vi "HWhist-SingleCurve.vi"() -> ()   [LabVIEW 2023]
doc: "This example demonstrates how to use the Becker&Hickl LV wrappers to acquire single decay curves in a continuous loop.\nThe SPC parameters can be adjusted during the run. The rates and status flags are continuously updated.\nIt is also possible to save the acquired data to a SDT or CSV file.\nClick this window's red X to stop this VI.\n\ninfo@becker-hickl.com"
uses:
  SPC_Wrappers/SPC_Controls/ConfigMem.ctl
  Example_Controls/UserInput.ctl
  SPC_Wrappers/SPC_Controls/SPC_RatesCluster.ctl
  SPC_Wrappers/SPC_Controls/ADCResolution.ctl
  SPC_Wrappers/SPC_Controls/ModuleType.ctl
  SPC_Wrappers/SPC_Controls/SPCdata.ctl
  SPC_Wrappers/SPC_Controls/StateCluster.ctl
  SPC_Wrappers/SPC_Controls/dither_range.ctl
  SPC_Wrappers/SPC_Controls/macro_time_clk.ctl
  <vilib>/Utility/file.llb/Write Delimited Spreadsheet (I64).vi
panel:
  in  "Page":i16(ring) caption="Use Page No" items=["0", "1", "2", "3", "4", "5", "6", "7", "8", "9", "10", "11", "12", "13", "14", "15"]
  in  "Init":bool
  out "SPC_StateCluster":T1
  out "SPCdata":T2
  in  "TO":i32=-1
  in  "Module Type":T3=150 items=["SPC-600"=600, "SPC-630"=630, "SPC-700"=700, "SPC-730"=730, "SPC-130"=130, "SPC-830"=830, "SPC-140"=140, "SPC-930"=930, "DPC-230"=230, "SPC-150"=150, "SPC-150 N"=151, "SPC-150 NX"=152, "SPC-130 EM"=131, "SPC-130 EMN"=132, "SPC-130IN"=135, "SPC-130INX"=136, "SPC-130INXX"=137, "SPC-160"=160, "SPC-160 X"=161, "SPC-160 PCIE"=162, "SPC-180 N"=180, "SPC-180 NX"=181, "SPC-180 NXX"=182, "SPC-180 N-USB"=185, "SPC-180 NX-USB"=186, "SPC-180 NXX-USB"=187, "SPC-QC-104"=104, "SPC-QC-004"=4, "SPC-QC-106"=106, "DPC-330"=330, "PMS-800"=800, "SPC-590"=590, "Simulation"=-1]
  out "Serial Number":string="3F0668"
  in  "RepeatMeas":bool
  in  "SingleMeas":bool
  out "DLL Path":path=path "C:/Program Files (x86)/BH/SPCM/DLL/spcm32x64.dll"
  out "Data":u16[][](graph)
  in  "Save Data As":enum32{"SDT", "CSV"}(radio)
  in  "No of Routing Channels":i16(ring)=1 items=["1"=1, "2"=2, "3"=3, "4"=4, "5"=5, "6"=6, "7"=7, "8"=8, "9"=9, "10"=10, "11"=11, "12"=12, "13"=13, "14"=14, "15"=15, "16"=16]
  in  "ADC Resolution":T4=12 items=["1"=0, "4"=2, "16"=4, "64"=6, "256"=8, "1024"=10, "4096"=12]
  out "Mod No":i16
  out "Sync OK":bool=TRUE
  out "SPC_RatesCluster":T5={"Sync"=49999360.0, "CFD"=1709808.0, "TAC"=1444208.0, "ADC"=998080.0} {"Sync" scale=0.0..6000000.0; "ADC" scale=0.0..1000000.0; "TAC" scale=0.0..1000000.0; "CFD" scale=0.0..1000000.0}
  in  "User Input":T6={"tac_range"=50.0, "tac_gain"=3, "tac_offset"=12.0, "tac_limit_high"=96.0, "tac_limit_low"=3.0, "collect_time"=2.0, "sync_threshold"=-71.0, "sync_zc_level"=-5.0, "sync_freq_div"=1, "cfd_limit_low"=-50.0, "cfd_zc_level"=9.8} {"sync_freq_div" items=["1"=1, "2"=2, "4"=4]; "cfd_zc_level" min=-96 max=96 step=0.1 format="%#_3g"; "cfd_limit_low" min=-500 max=0 step=0.1 format="%#_3g"; "sync_zc_level" min=-96 max=96 step=0.1 format="%#_3g"; "sync_threshold" min=-500 max=-20 step=0.1 format="%#_3g"; "tac_limit_low" format="%.3g"; "tac_limit_high" min=0 max=100 step=0.1 format="%.3g"; "collect_time" min=1e-07 max=100000 step=0.001; "tac_offset" min=0 max=100 step=0.1 format="%.4g"; "tac_gain" min=1 max=15 step=1; "tac_range" format="%^#_6g"}
  in  "SaveData":bool
  in  "Name Of File":string="HW-SingleDecay"
  in  "SavingFolder":path=path "C:/temp"
  out "SPC memory config":T7={"Max Block No"=16384, "Blocks Per Frame"=1, "Frames Per Page"=1, "Maxpage"=16384, "Block Length"=256} {"Frames Per Page" min=1 step=1; "Maxpage" min=1; "Blocks Per Frame" min=1 step=1}
  in  "StopVi":bool=TRUE
  # "This example demonstrates how to use the Becker&Hickl LV wrappers to acquire single decay curves in a continuous loop.\nThe SPC parameters can be adjusted during the run. The rates and status flags are continuously updated.\nIt is also possible to save the acquired data to a SDT or CSV file.\nClick this window's red X to stop this VI."
  # "See Tip-Strip for details"
  # "(c) 2023 Becker & Hickl GmbH\n     ALL RIGHTS RESERVED."
  # "TAC / Time Range"
  # "CFD"
  # "(start)"
  # "SYNC"
  # "(stop)"
  # "range"
  # "gain"
  # "threshold(LL)"
  # "offset"
  # "limit high"
  # "limit low"
  # "zero cross(ZC)"
  # "Collection Time"
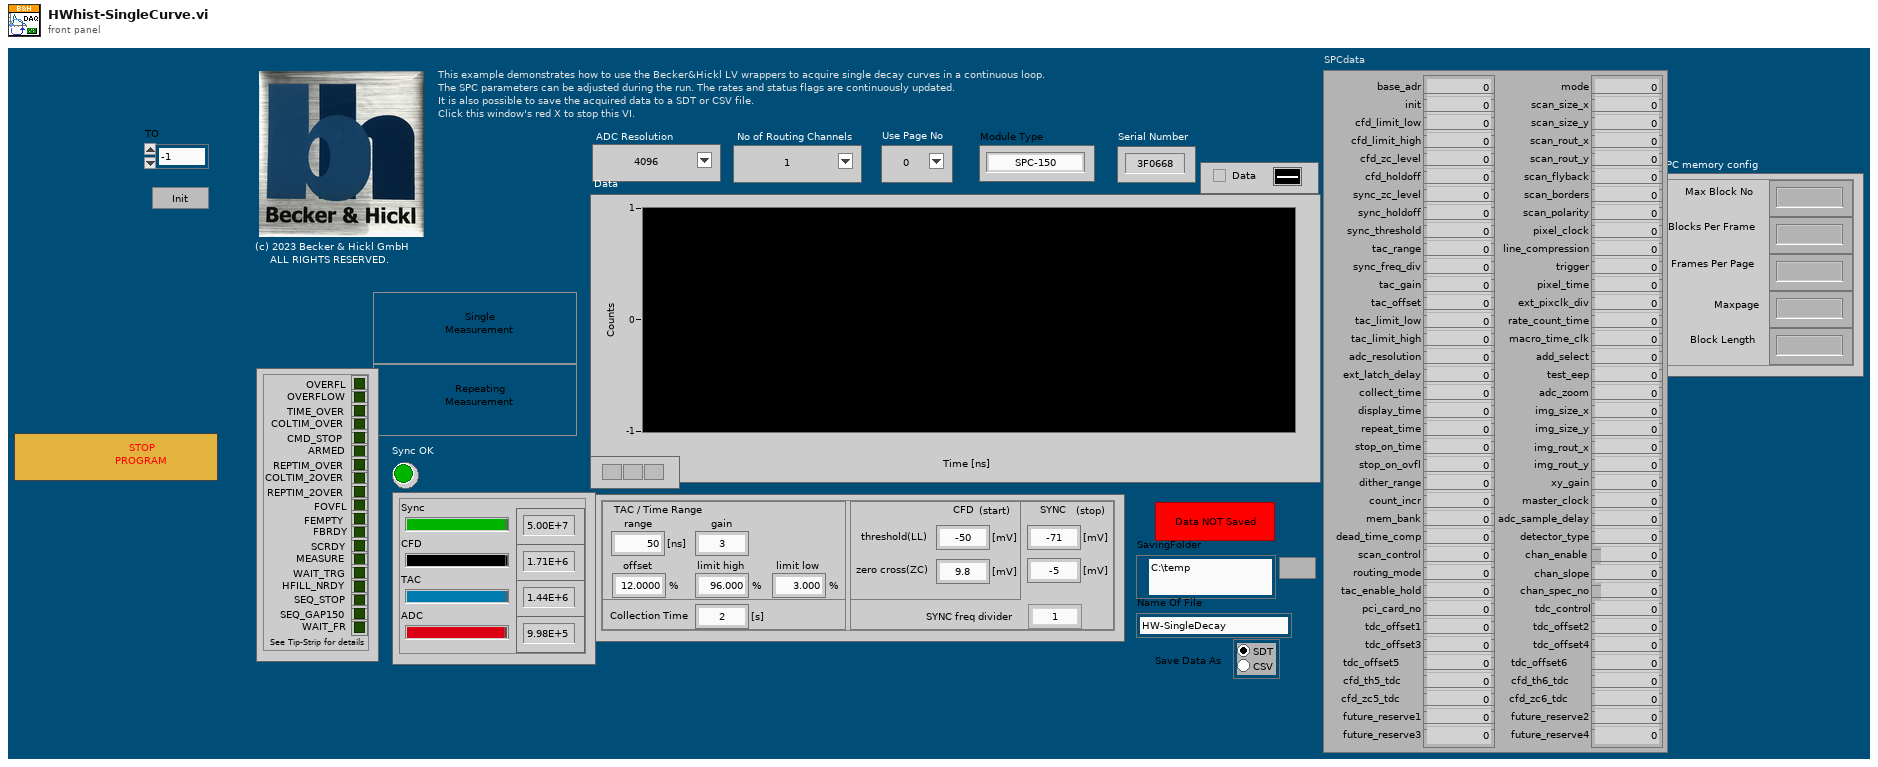
[diagram p1: front panel]
types:
  T1 = typedef "StateCluster.ctl" = cluster{"OVERFL":bool, "OVERFLOW":bool, "TIME_OVER":bool, "COLTIM_OVER":bool, "CMD_STOP":bool, "ARMED":bool, "REPTIM_OVER":bool, "COLTIM_2OVER":bool, "REPTIM_2OVER":bool, "FOVFL":bool, "FEMPTY":bool, "FBRDY":bool, "SCRDY":bool, "MEASURE":bool, "WAIT_TRG":bool, "HFILL_NRDY":bool, "SEQ_STOP":bool, "SEQ_GAP150":bool, "WAIT_FR":bool}
  T2 = typedef "SPCdata.ctl" = cluster{"base_adr":u16, "init":i16, "cfd_limit_low":sgl, "cfd_limit_high":sgl, "cfd_zc_level":sgl, "cfd_holdoff":sgl, "sync_zc_level":sgl, "sync_holdoff":sgl, "sync_threshold":sgl, "tac_range":sgl, "sync_freq_div":i16, "tac_gain":i16, "tac_offset":sgl, "tac_limit_low":sgl, "tac_limit_high":sgl, "adc_resolution":i16, "ext_latch_delay":i16, "collect_time":sgl, "display_time":sgl, "repeat_time":sgl, "stop_on_time":i16, "stop_on_ovfl":i16, "dither_range":i16, "count_incr":i16, "mem_bank":i16, "dead_time_comp":i16, "scan_control":u16, "routing_mode":u16, "tac_enable_hold":sgl, "pci_card_no":i16, "mode":u16, "scan_size_x":u32, "scan_size_y":u32, "scan_rout_x":u32, "scan_rout_y":u32, "scan_flyback":u32, "scan_borders":u32, "scan_polarity":u16, "pixel_clock":u16, "line_compression":u16, "trigger":u16, "pixel_time":sgl, "ext_pixclk_div":u32, "rate_count_time":sgl, "macro_time_clk":i16, "add_select":i16, "test_eep":i16, "adc_zoom":i16, "img_size_x":u32, "img_size_y":u32, "img_rout_x":u32, "img_rout_y":u32, "xy_gain":i16, "master_clock":i16, "adc_sample_delay":i16, "detector_type":i16, "chan_enable":u32, "chan_slope":u32, "chan_spec_no":u32, "tdc_control":u32, "tdc_offset1":sgl, "tdc_offset2":sgl, "tdc_offset3":sgl, "tdc_offset4":sgl, "tdc_offset5":sgl, "tdc_offset6":sgl, "cfd_th5_tdc":sgl, "cfd_th6_tdc":sgl, "cfd_zc5_tdc":sgl, "cfd_zc6_tdc":sgl, "future_reserve1":u64, "future_reserve2":u64, "future_reserve3":u64, "future_reserve4":u64}
  T3 = typedef "ModuleType.ctl" = i16
  T4 = typedef "ADCResolution.ctl" = i16
  T5 = typedef "SPC_RatesCluster.ctl" = cluster{"Sync":sgl, "CFD":sgl, "TAC":sgl, "ADC":sgl}
  T6 = typedef "UserInput.ctl" = cluster{"tac_range":sgl, "tac_gain":i16, "tac_offset":sgl, "tac_limit_high":sgl, "tac_limit_low":sgl, "collect_time":sgl, "sync_threshold":sgl, "sync_zc_level":sgl, "sync_freq_div":i16, "cfd_limit_low":sgl, "cfd_zc_level":sgl}
  T7 = typedef "ConfigMem.ctl" = cluster{"Max Block No":i32, "Blocks Per Frame":i32, "Frames Per Page":i32, "Maxpage":i32, "Block Length":i32}
  T8 = typedef "macro_time_clk.ctl" = enum16{"25ns", "Sync", "1/2 Sync", "1/4 Sync", "1/8 Sync"}
  T9 = typedef "dither_range.ctl" = i16
  T10 = enum8{"Enabled", "Disabled", "Disabled and Grayed Out"}
  T11 = typedef "SPCModInfo.ctl" = cluster{"Module Type":T3, "Bus Number":i16, "Slot Number":i16, "in Use":i16, "Init Status":i16, "Base I/O Addr":u16}
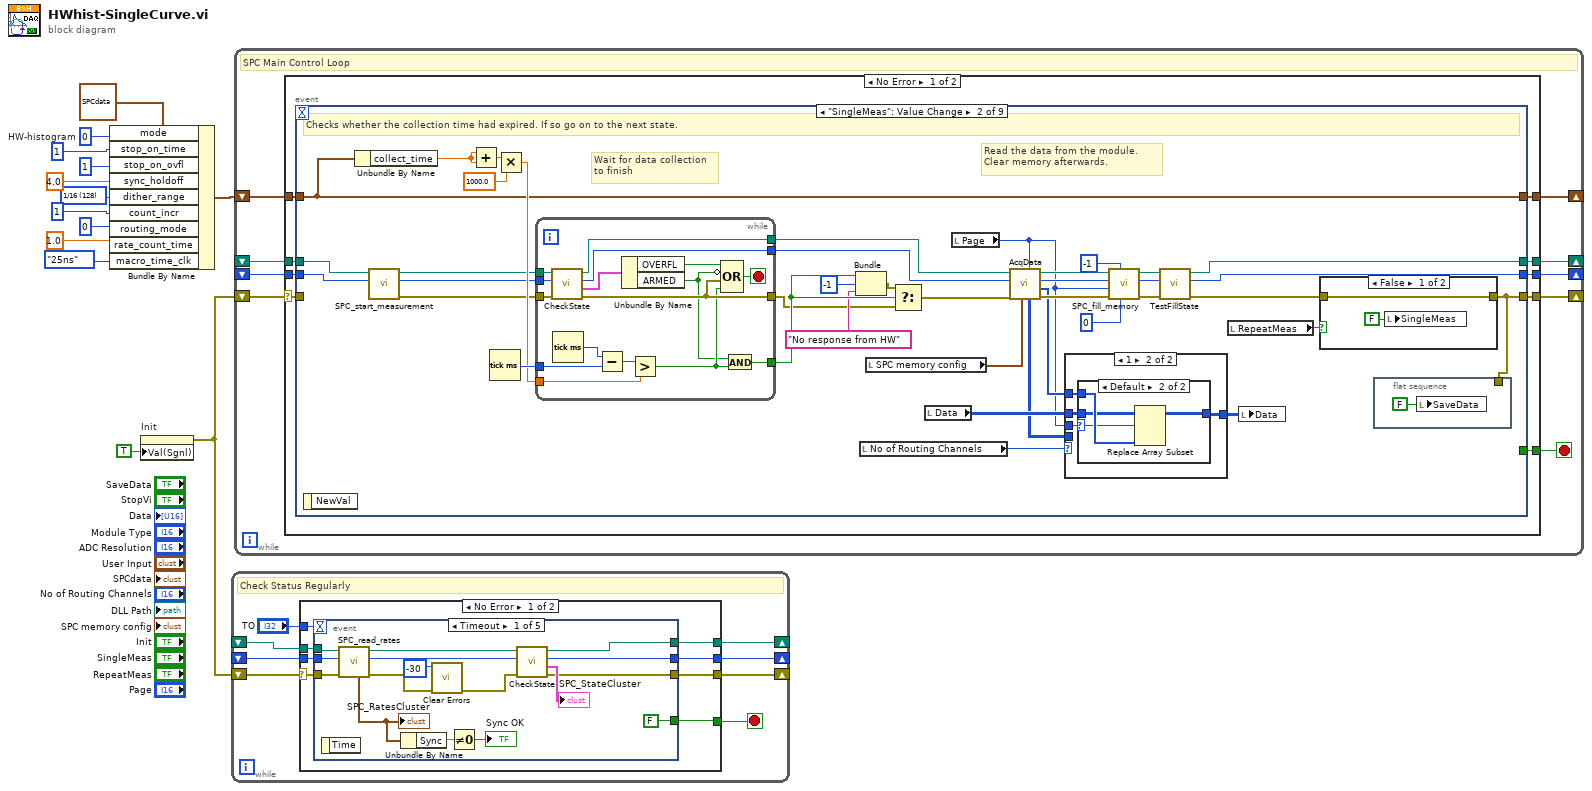
[diagram p0: block diagram]
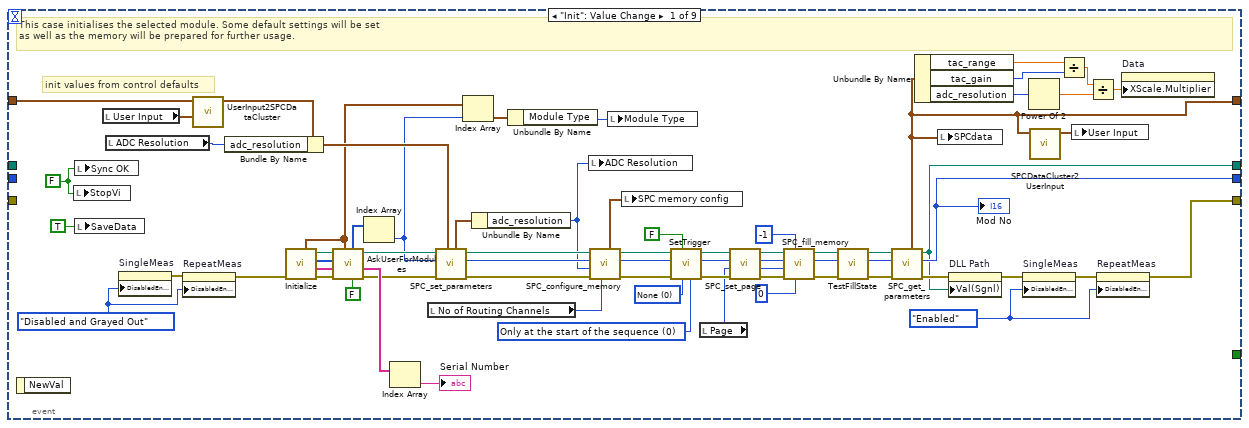
[diagram p2: hidden frame]
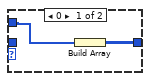
[diagram p4: hidden frame]
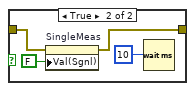
[diagram p5: hidden frame]
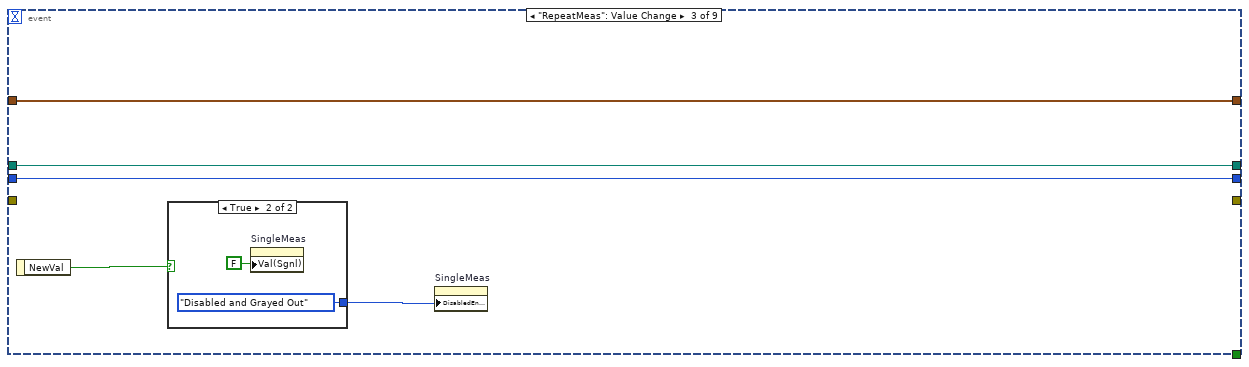
[diagram p6: hidden frame]
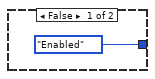
[diagram p7: hidden frame]
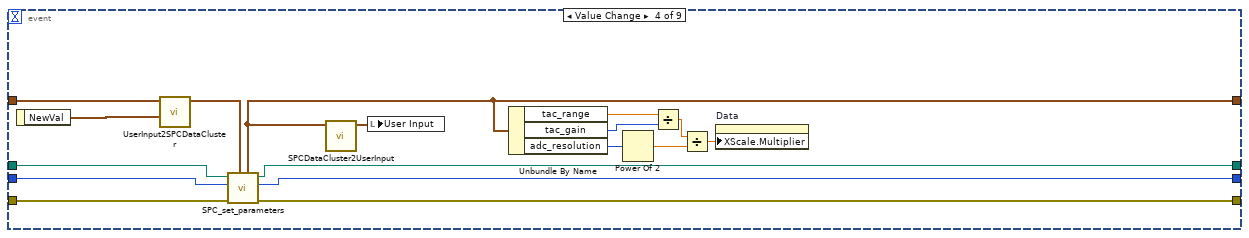
[diagram p8: hidden frame]
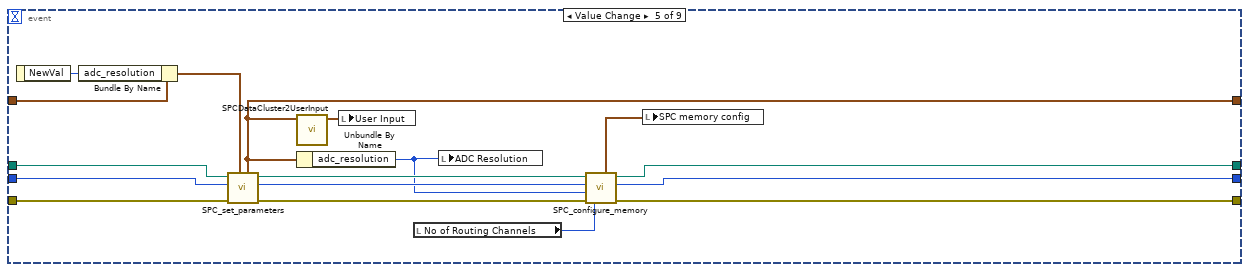
[diagram p9: hidden frame]
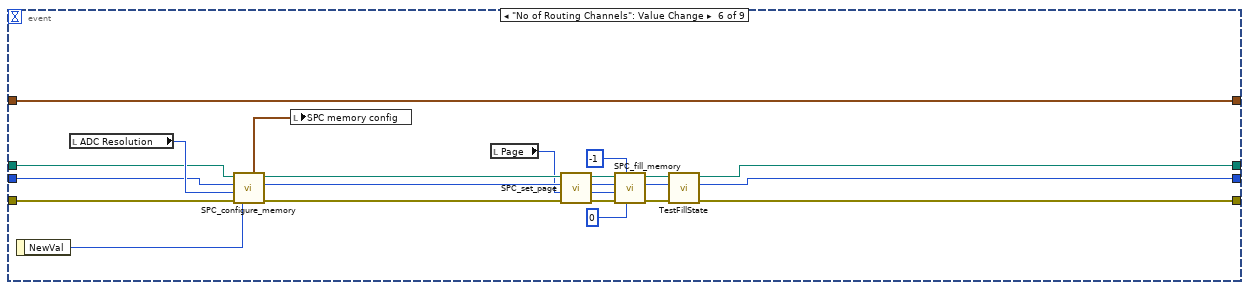
[diagram p10: hidden frame]
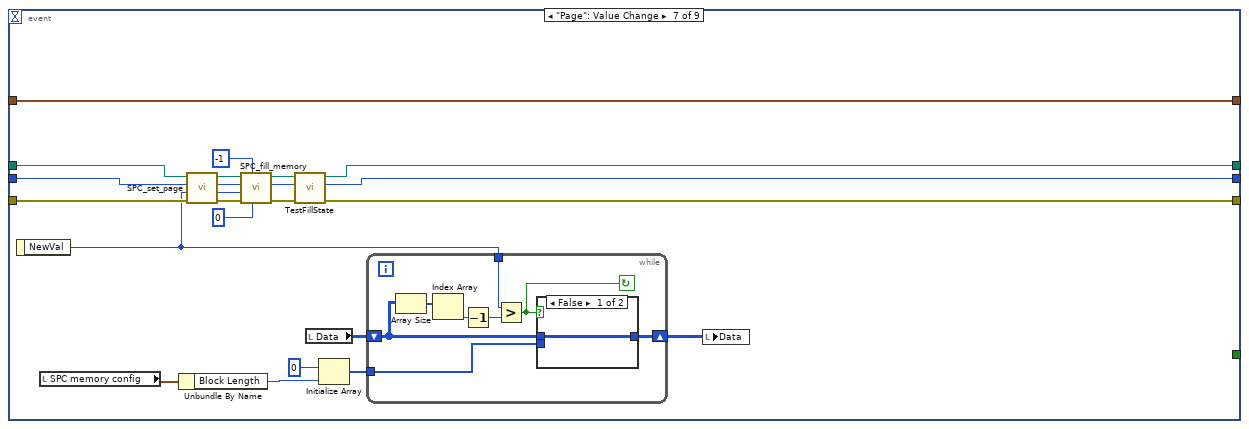
[diagram p11: hidden frame]
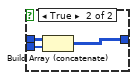
[diagram p12: hidden frame]
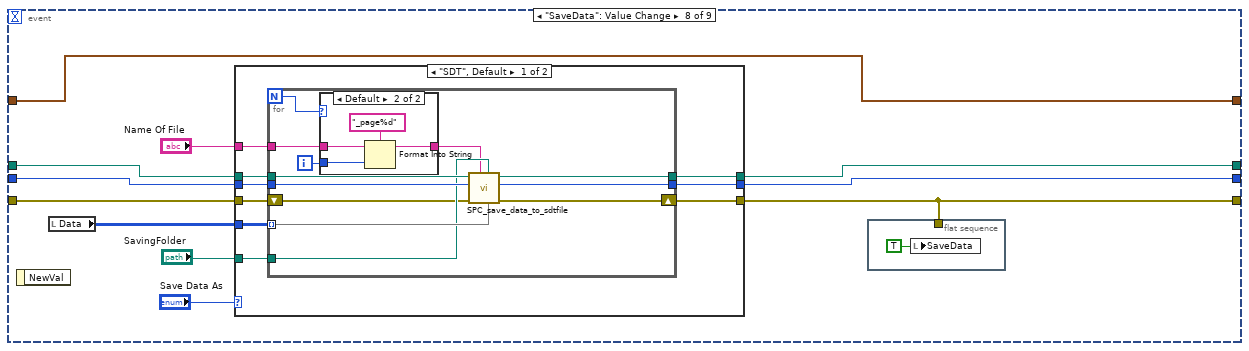
[diagram p13: hidden frame]
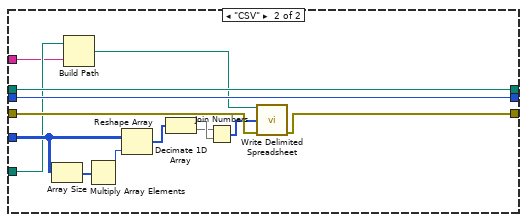
[diagram p15: hidden frame]
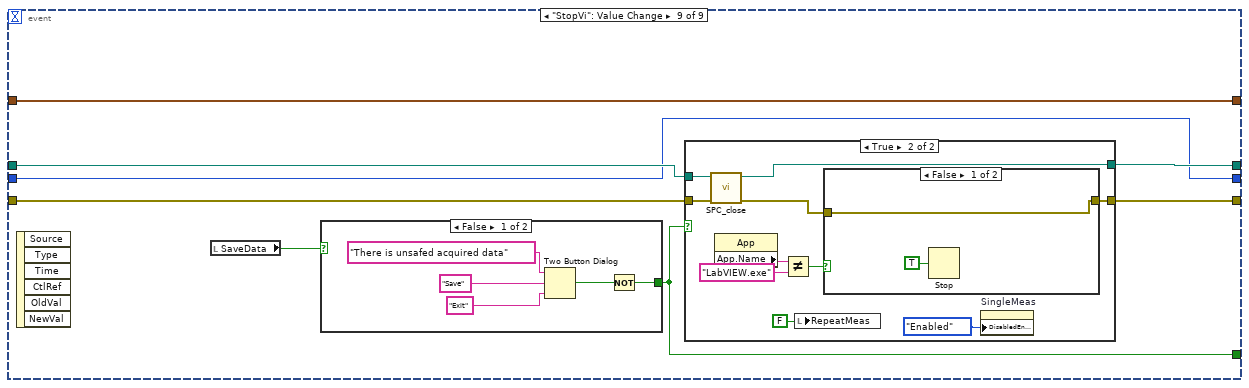
[diagram p16: hidden frame]
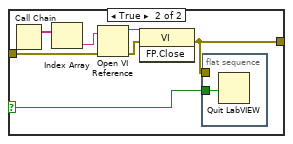
[diagram p18: hidden frame]
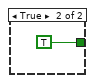
[diagram p19: hidden frame]
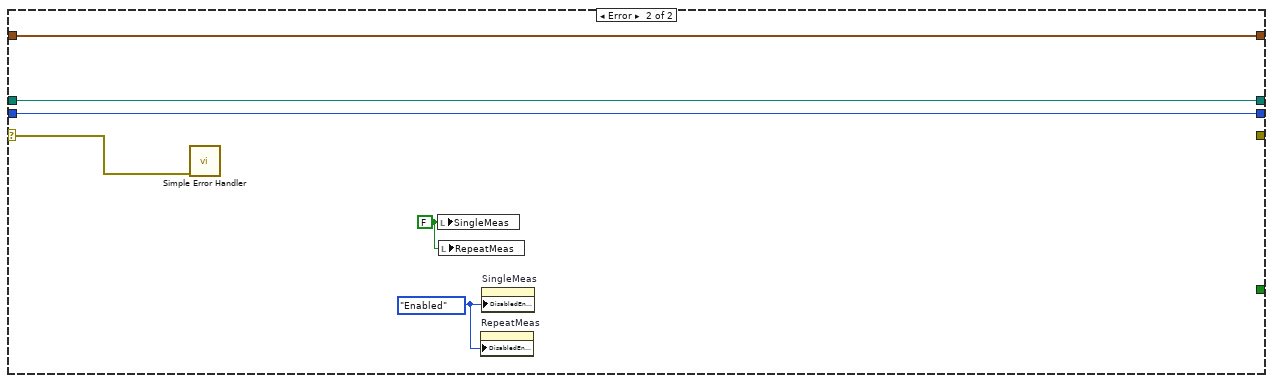
[diagram p20: hidden frame]
diagram:
  w2 = T9 128 items=["0"=0, "1/64"=32, "1/32"=64, "1/16"=128, "1/8"=256] ("DithRange")
  w4 = u16 0  # HW-histogram
  n1 = Bundle By Name(cluster=T2 {"base_adr"=896, "init"=0, "cfd_limit_low"=5.0, "cfd_limit_high"=80.0, "cfd_zc_level"=0.0, "cfd_holdoff"=5.0, "sync_zc_level"=0.0, "sync_holdoff"=4.0, "sync_threshold"=-20.0, "tac_range"=50.0, "sync_freq_div"=1, "tac_gain"=1, "tac_offset"=0.0, "tac_limit_low"=10.0, "tac_limit_high"=80.0, "adc_resolution"=10, "ext_latch_delay"=0, "collect_time"=0.01, "display_time"=1.0, "repeat_time"=10.0001, "stop_on_time"=1, "stop_on_ovfl"=1, "dither_range"=0, "count_incr"=1, "mem_bank"=0, "dead_time_comp"=1, "scan_control"=61440, "routing_mode"=0, "tac_enable_hold"=10.0, "pci_card_no"=-1, "mode"=0, "scan_size_x"=1, "scan_size_y"=1, "scan_rout_x"=1, "scan_rout_y"=1, "scan_flyback"=0, "scan_borders"=0, "scan_polarity"=0, "pixel_clock"=0, "line_compression"=1, "trigger"=0, "pixel_time"=5e-08, "ext_pixclk_div"=1, "rate_count_time"=1.0, "macro_time_clk"=0, "add_select"=0, "test_eep"=0, "adc_zoom"=0, "img_size_x"=1, "img_size_y"=1, "img_rout_x"=1, "img_rout_y"=1, "xy_gain"=1, "master_clock"=0, "adc_sample_delay"=0, "detector_type"=1, "chan_enable"=4191231, "chan_slope"=0, "chan_spec_no"=34835, "tdc_control"=0, "tdc_offset1"=0.0, "tdc_offset2"=0.0, "tdc_offset3"=0.0, "tdc_offset4"=0.0, "tdc_offset5"=0.0, "tdc_offset6"=0.0, "cfd_th5_tdc"=0.0, "cfd_th6_tdc"=0.0, "cfd_zc5_tdc"=0.0, "cfd_zc6_tdc"=0.0, "future_reserve1"=0, "future_reserve2"=0, "future_reserve3"=0, "future_reserve4"=0} ("SPCdata In"), "mode"=w4, "stop_on_time"=i16 1 ("Stop on Time"), "stop_on_ovfl"=i16 1 ("Stop on Overflow"), "sync_holdoff"=sgl 4.0, "dither_range"=w2, "count_incr"=i16 1 ("Count Increment"), "routing_mode"=u16 0 ("Routing Mode"), "rate_count_time"=sgl 1.0 ("CFD ZC Level [mV]"), "macro_time_clk"=macro_time_clk."25ns") -> (w13:T2)
  n2 = property on="Init" class="Bool (strict)"("Val(Sgnl)"=TRUE ("Value (Signaling)")) -> (error out=w6:errorcluster)  [unwired: 2 in, 1 out]
  n3 = while {
    shift-right: [w20] -> _
    shift-left: w6 -> [w21]
    shift-right: [w17] -> _
    shift-left: _ -> [w18]
    shift-right: [w15] -> _
    shift-left: _ -> [w19]
    stop <- w14 stop-if-true
    # "Check Status Regularly"
    n4 = case shown="No Error" w21 {
      selector: w21 -> [w29 w63]
      tunnel: [w28 _] -> w20
      tunnel: w19 -> [w27 w66]
      tunnel: w18 -> [w26 w67]
      tunnel: [w25 w67] -> w17
      tunnel: "TO" -> [w24 _]
      tunnel: [w23 w66] -> w15
      tunnel: [w22 _] -> w14
      frame No Error {
        n5 = event shown="[0] Timeout" {
          selector: _ -> [_ _ _ _ _]
          dyn-events: _ -> [_ _ _ _ _]
          timeout: w24 -> [_ _ _ _ _]
          tunnel: w29 -> [w43 w52 _ _ _]
          tunnel: [w35 w51 _ _ _] -> w28
          tunnel: w27 -> [w40 _ _ _ _]
          tunnel: w26 -> [w39 _ _ _ _]
          tunnel: [w31 w48 _ _ _] -> w25
          tunnel: [w34 w47 _ _ _] -> w23
          tunnel: [FALSE ("Sync OK") _ _ _ _] -> w22
          event Timeout {
            n6 = event-data() -> ()  [unwired: 1 in, 1 out]
            n7 = call "SPC_read_rates.vi"("Error In"=w43, "Module No"=w40, "DLL Path"=w39) -> ("Error Out"=w45:errorcluster, "Module No"=w33:i16, "DLL Path"=w32:path, "SPC_RatesCluster"=w30:T5)  [unwired: 5 in]
            "SPC_RatesCluster" <- w30
            n8 = Unbundle By Name(w30) -> ("Sync"=w41:sgl)
            n9 = call <vilib>:"Clear Errors.vi"("error in (no error)"=w45, "specific error code to clear (0: all)"=-30) -> ("error out"=w36:errorcluster)  [unwired: 4 in, 1 out]
            n10 = Not Equal To 0?(x=w41) -> (x != 0?=→"Sync OK":bool)
            n11 = call "CheckState.vi"("Error In"=w36, "Module No."=w33, "DLL Path"=w32) -> ("Error Out"=w35:errorcluster, "SPC_StateCluster"=→"SPC_StateCluster":T1, "Module No."=w34:i16, "DLL Path"=w31:path)  [unwired: 4 in, 1 out]
          }
          event "DLL Path": Value Change {
            n12 = event-data() -> ("NewVal"=w49:path)  [unwired: 1 in]
            n13 = local read "Mod No"() -> (w50:i16)
            n14 = call "SPC_clear_rates.vi"("Error In"=w52, "Module no"=w50, "DLL Path"=w49) -> ("Error Out"=w51:errorcluster, "Module  No"=w47:i16, "DLL Path"=w48:path)  [unwired: 6 in]
            n15 = local write "TO"(1100 ("milliseconds to wait")) -> ()
          }
          event Application Instance Close? {
            n16 = event-data() -> ()  [unwired: 1 in, 1 out]
            n17 = property on="StopVi" class="Bool (strict)"("Val(Sgnl)"=TRUE ("Value (Signaling)")) -> ()  [unwired: 2 in, 2 out]
            n18 = event-data("Discard?"=TRUE) -> ()  [unwired: 2 in, 1 out]
          }
          event Panel Close? {
            n19 = event-data() -> ()  [unwired: 1 in, 1 out]
            n20 = property on="StopVi" class="Bool (strict)"("Val(Sgnl)"=TRUE ("Value (Signaling)")) -> ()  [unwired: 2 in, 2 out]
            n21 = event-data("Discard?"=TRUE) -> ()  [unwired: 1 in, 1 out]
          }
          event Menu Selection? (App) {
            n22 = event-data() -> ("ItemTag"=w57:string)  [unwired: 1 in]
            n23 = case shown="\"APP_CLOSE\", \"APP_EXIT\", \"APP_STOP\"" w57 {
              frame Default {
                # "nothing to deal with"
              }
              frame "APP_CLOSE", "APP_EXIT", "APP_STOP" {
                n24 = property on="StopVi" class="Bool (strict)"("Val(Sgnl)"=TRUE ("Value (Signaling)")) -> ()  [unwired: 2 in, 2 out]
              }
            }
            n25 = event-data("Discard?"=TRUE) -> ()  [unwired: 1 in, 1 out]
          }
        }
      }
      frame Error {
        # "Stop the SPC main control\nloop if an errors occurs"
        n26 = call <vilib>:"Clear Errors.vi"("error in (no error)"=w63, "specific error code to clear (0: all)"=-33) -> ("error out"=w64:errorcluster)  [unwired: 4 in, 1 out]
        n27 = call <vilib>:"Simple Error Handler.vi"("error in (no error)"=w64) -> ("error out"=w61:errorcluster)  [unwired: 4 in, 4 out]
        n28 = call <vilib>:"Clear Errors.vi"("error in (no error)"=w61) -> ("error out"=w60:errorcluster)  [unwired: 5 in, 1 out]
        n29 = property on="StopVi" class="Bool (strict)"(error in=w60, "Val(Sgnl)"=TRUE ("Value (Signaling)")) -> ()  [unwired: 1 in, 2 out]
      }
    }
  }
  n30 = while {
    shift-right: [w69] -> _
    shift-left: w6 -> [w74]
    shift-right: [w75] -> _
    shift-left: _ -> [w72]
    shift-right: [w71] -> _
    shift-left: _ -> [w73]
    shift-right: [w70] -> _
    shift-left: w13 -> [w76]
    stop <- w68 stop-if-true
    # "SPC Main Control Loop"
    n31 = case shown="No Error" w74 {
      selector: w74 -> [w83 w420]
      tunnel: w76 -> [w85 w417]
      tunnel: [w84 w418] -> w75
      tunnel: w73 -> [w82 w419]
      tunnel: w72 -> [w81 w418]
      tunnel: [w80 w419] -> w71
      tunnel: [w79 w417] -> w70
      tunnel: [w78 _] -> w69
      tunnel: [w77 _] -> w68
      frame No Error {
        n32 = event shown="[1] \"SingleMeas\": Value Change" {
          selector: _ -> [_ _ _ _ _ _ _ _ _]
          dyn-events: _ -> [_ _ _ _ _ _ _ _ _]
          timeout: _ -> [_ _ _ _ _ _ _ _ _]
          tunnel: w85 -> [w90 w183 w229 w244 w263 w285 w296 w337 w386]
          tunnel: [w107 w163 w228 w251 w258 w272 w302 w333 w383] -> w84
          tunnel: w83 -> [_ _ _ w247 w267 w286 w301 w336 w384]
          tunnel: w82 -> [_ w180 w227 w246 w266 w287 w305 w331 w379]
          tunnel: w81 -> [_ w181 w228 w245 w265 w288 w303 w332 w382]
          tunnel: [w116 w162 w227 w249 w260 w271 w304 w334 w379] -> w80
          tunnel: [w110 w183 w229 w235 w254 w285 w296 w337 w386] -> w79
          tunnel: [w118 w154 _ w250 w261 w270 w300 w335 w381] -> w78
          tunnel: [_ _ _ _ _ _ _ _ w380] -> w77
          event "Init": Value Change {
            w109 = T10."Disabled and Grayed Out" ("Disabled")
            w126 = T10."Enabled" ("Disabled")
            w131 = FALSE
            w132 = i16 0 items=["Only at the start of the sequence"=0, "On each bank"=256, "On each curve in the bank"=768] ("Start Trigger")
            w134 = i16 0 items=["None", "Falling Edge", "Rising Edge"] ("Ext. Trigger Condition")
            # "init values from control defaults"
            # "This case initialises the selected module. Some default settings will be set\nas well as the memory will be prepared for further usage."
            n33 = event-data() -> ()  [unwired: 1 in, 1 out]
            n34 = local write "StopVi"(w131) -> ()
            n35 = local write "Sync OK"(w131) -> ()
            n36 = local write "SaveData"(TRUE ("SaveData")) -> ()
            n37 = local read "User Input"() -> (w88:T6)
            n38 = local read "ADC Resolution"() -> (w99:T4)
            n39 = property on="SingleMeas" class="Bool (strict)"("DisabledEnum"=w109) -> (error out=w125:errorcluster)  [unwired: 2 in, 1 out]
            n40 = property on="RepeatMeas" class="Bool (strict)"(error in=w125, "DisabledEnum"=w109) -> (error out=w124:errorcluster)  [unwired: 1 in, 1 out]
            n41 = call "UserInput2SPCDataCluster.vi"("UserInput_In"=w88, "SPCData_In"=w90) -> ("SPCData_Out"=w89:T2)  [unwired: 9 in]
            n42 = Bundle By Name(cluster=w89, "adc_resolution"=w99) -> (w100:T2)
            n43 = call "Initialize.vi"("ErrorIn"=w124) -> ("ErrorOut"=w144:errorcluster, "SerialNumbersArray"=w143:string[], "ModuleNoArray"=w138:i16[], "DLL Path"=w108:path, "SPCModulesArray"=w93:T11[])  [unwired: 6 in]
            n44 = call "AskUserForModules.vi"("MultiModule"=FALSE, "SPCModulesArray"=w93, "Error In"=w144, "Serial Number"=w143, "ModuleNoArray"=w138, "DLL Path"=w108) -> ("Error Out"=w102:errorcluster, "ActiveSerialNumbers"=w122:string[], "DLL Path"=w105:path, "ActiveModuleNo"=w142:i16[])  [unwired: 1 in, 1 out]
            n45 = Index Array(array=w142) -> (element=w92:i16)  [unwired: 1 in]
            n46 = Index Array(array=w122) -> (element=→"Serial Number":string)  [unwired: 1 in]
            n47 = local read "No of Routing Channels"() -> (w119:i16)
            n48 = call "SPC_set_parameters.vi"("SPCdata In"=w100, "Error In"=w102, "Module No."=w92, "DLL Path"=w105) -> ("Error Out"=w101:errorcluster, "Module No"=w103:i16, "DLL Path"=w104:path, "SPCdata Out"=w95:T2)  [unwired: 4 in]
            n49 = Index Array(array=w93, index=w92) -> (element=w121:T11)
            n50 = Unbundle By Name(w95) -> ("adc_resolution"=w94:i16)
            n51 = Unbundle By Name(w121) -> ("Module Type"=w120:T3)
            n52 = local write "ADC Resolution"(w94) -> ()
            n53 = call "SPC_configure_memory.vi"("No of Routing\nChannels"=w119, "Error In"=w101, "ADC Resolution [exponent]"=w94, "Module No"=w103, "DLL Path"=w104) -> ("Error Out"=w96:errorcluster, "Module No"=w97:i16, "DLL Path"=w98:path, "SPCMemConfig"=w106:T7)  [unwired: 2 in, 1 out]
            n54 = local write "Module Type"(w120) -> ()
            n55 = local write "SPC memory config"(w106) -> ()
            n56 = call "SetTrigger.vi"("Start Trigger"=w132, "Ext. Trigger Condition"=w134, "Master"=FALSE ("Master/Slave?"), "Error In"=w96, "Module No"=w97, "DLL Path"=w98) -> ("Error Out"=w136:errorcluster, "Module No"=w135:i16, "DLL Path"=w137:path)  [unwired: 3 in]
            n57 = local read "Page"() -> (w86:i16)
            n58 = call "SPC_set_page.vi"("Error In"=w136, "Page"=w86, "Module No"=w135, "DLL Path"=w137) -> ("Error Out"=w147:errorcluster, "Page"=w153:i32, "Module No"=w148:i16, "DLL Path"=w149:path)  [unwired: 4 in]
            n59 = call "SPC_fill_memory.vi"("Fill Value"=u16 0 ("Fill value"), "Block to be Filled"=-1 ("Block to be filled"), "Error In"=w147, "Page"=w153, "Module No"=w148, "DLL Path"=w149) -> ("Error Out"=w150:errorcluster, "Module No"=w151:i16, "DLL Path"=w152:path)  [unwired: 2 in, 1 out]
            n60 = call "TestFillState.vi"("Error In"=w150, "Module No"=w151, "DLL Path"=w152) -> ("Error Out"=w139:errorcluster, "Module No"=w140:i16, "DLL Path"=w141:path)  [unwired: 6 in]
            n61 = call "SPC_get_parameters.vi"("Error In"=w139, "Module No"=w140, "DLL Path"=w141) -> ("Error Out"=w130:errorcluster, "Module No"=w116:i16, "DLL Path"=w107:path, "SPCdata"=w110:T2)  [unwired: 5 in]
            "Mod No" <- w116
            n62 = Unbundle By Name(w110) -> ("tac_range"=w114:sgl, "tac_gain"=w113:i16, "adc_resolution"=w112:i16)
            n63 = local write "SPCdata"(w110) -> ()
            n64 = property on="DLL Path" class="Path"(error in=w130, "Val(Sgnl)"=w107) -> (error out=w128:errorcluster)  [unwired: 1 in, 1 out]
            n65 = property on="SingleMeas" class="Bool (strict)"(error in=w128, "DisabledEnum"=w126) -> (error out=w127:errorcluster)  [unwired: 1 in, 1 out]
            n66 = Power Of 2(x=w112) -> (2^x=w111:dbl)
            n67 = call "SPCDataCluster2UserInput.vi"("SPCdata In"=w110) -> ("UserInput Out"=w123:T6)  [unwired: 10 in]
            n68 = Divide(x=w114, y=w113) -> (x/y=w115:sgl)
            n69 = local write "User Input"(w123) -> ()
            n70 = Divide(x=w115, y=w111) -> (x/y=w91:dbl)
            n71 = property on="RepeatMeas" class="Bool (strict)"(error in=w127, "DisabledEnum"=w126) -> (error out=w118:errorcluster)  [unwired: 1 in, 1 out]
            n72 = property on="Data" class="WFGraph (strict)"("XScale.Multiplier"=w91) -> ()  [unwired: 2 in, 2 out]
          }
          event "SingleMeas": Value Change {
            # "Wait for data collection\nto finish"
            # "Read the data from the module.\nClear memory afterwards."
            # "Checks whether the collection time had expired. If so go on to the next state."
            n73 = event-data() -> ()  [unwired: 1 in, 1 out]
            n74 = Unbundle By Name(w183) -> ("collect_time"=w161:sgl)
            n75 = call "SPC_start_measurement.vi"("Module No"=w180, "DLL Path"=w181) -> ("Error Out"=w182:errorcluster, "Module No"=w179:i16, "DLL Path"=w178:path)  [unwired: 7 in]
            n76 = Add(x=w161, y=w161) -> (x+y=w186:sgl)
            n77 = Tick Count (ms)() -> (millisecond timer value=w192:u32)
            n78 = Multiply(x=w186, y=sgl 1000.0) -> (x*y=w185:sgl)
            n79 = while {
              tunnel: w178 -> [w226]
              tunnel: w179 -> [w225]
              tunnel: w182 -> [w224]
              tunnel: [w221] -> w167
              tunnel: [w220] -> w166
              tunnel: [w219] -> w187
              tunnel: w192 -> [w216]
              tunnel: [w212] -> w190
              tunnel: w185 -> [w213]
              stop <- w223 stop-if-true
              n80 = call "CheckState.vi"("Error In"=w224, "Module No."=w225, "DLL Path"=w226) -> ("Error Out"=w219:errorcluster, "SPC_StateCluster"=w222:T1, "Module No."=w220:i16, "DLL Path"=w221:path)  [unwired: 4 in, 1 out]
              n81 = Tick Count (ms)() -> (millisecond timer value=w217:u32)
              n82 = Subtract(x=w217, y=w216) -> (x-y=w215:u32)
              n83 = Unbundle By Name(w222) -> ("OVERFL"=w218:bool, "ARMED"=w211:bool)
              n84 = Greater?(x=w215, y=w213) -> (0:w214:bool)
              n85 = Compound Arithmetic op=OR(w218, invert w211, w219, w214) -> (w223:bool)
              n86 = And(x=w211, y=w214) -> (x .and. y?=w212:bool)
            }
            n87 = Bundle(w190, "Code"=-1, "Source"="No response from HW") -> (w191:cluster{bool, "Code":i32, "Source":string})  [unwired: 1 in]
            n88 = local read "No of Routing Channels"() -> (w157:i16)
            n89 = local read "SPC memory config"() -> (w169:T7)
            n90 = Select(t=w191, s=w190, f=w187) -> (s? t:f=w168:errorcluster)
            n91 = local read "Data"() -> (w158:u16[][])
            n92 = local read "Page"() -> (w155:i16)
            n93 = call "AcqData.vi"("Page No"=w155, "SPC Memory Config"=w169, "Error In"=w168, "Module No"=w166, "DLL Path"=w167) -> ("Error Out"=w172:errorcluster, "SingleBlockData"=w160:u16[], "Module No"=w170:i16, "DLL Path"=w171:path, "MultiBlockData"=w156:u16[][])  [unwired: 2 in]
            n94 = case shown="1" w157 {
              tunnel: w160 -> [_ w198]
              tunnel: [w194 w197] -> w159
              tunnel: w155 -> [_ w196]
              tunnel: w158 -> [_ w195]
              tunnel: w156 -> [w194 _]
              frame Default {
              }
              frame 1 {
                n95 = case shown="Default" w196 {
                  selector: w196 -> [_ w201]
                  tunnel: w198 -> [w199 w203]
                  tunnel: [w200 w204] -> w197
                  tunnel: w195 -> [_ w202]
                  frame 0 {
                    n96 = Build Array(w199) -> (w200:u16[][])
                  }
                  frame Default {
                    n97 = Replace Array Subset(array=w202, new element=w203, index (row)=w201) -> (w204:u16[][])  [unwired: 1 in]
                  }
                }
              }
            }
            n98 = call "SPC_fill_memory.vi"("Fill Value"=u16 0 ("Fill value"), "Block to be Filled"=-1 ("Block to be filled"), "Error In"=w172, "Page"=w155, "Module No"=w170, "DLL Path"=w171) -> ("Error Out"=w175:errorcluster, "Module No"=w176:i16, "DLL Path"=w177:path)  [unwired: 2 in, 1 out]
            n99 = call "TestFillState.vi"("Error In"=w175, "Module No"=w176, "DLL Path"=w177) -> ("Error Out"=w164:errorcluster, "Module No"=w162:i16, "DLL Path"=w163:path)  [unwired: 6 in]
            n100 = local read "RepeatMeas"() -> (w165:bool)
            n101 = local write "Data"(w159) -> ()
            n102 = case shown="False" w165 {
              tunnel: w164 -> [w206 w210]
              tunnel: [w206 w209] -> w154
              frame False {
                n103 = local write "SingleMeas"(FALSE ("StartMeas")) -> ()
              }
              frame True {
                n104 = property on="SingleMeas" class="Bool (strict)"(error in=w210, "Val(Sgnl)"=FALSE ("Value (Signaling)")) -> (error out=w209:errorcluster)  [unwired: 1 in, 1 out]
                n105 = Wait (ms)(milliseconds to wait=u32 10) -> ()  [unwired: 1 out]
              }
            }
            n106 = flat-sequence {
              tunnel: w154 -> [_]
              frame #0 {
                n107 = local write "SaveData"(FALSE ("SaveData")) -> ()
              }
            }
          }
          event "RepeatMeas": Value Change {
            n108 = event-data() -> ("NewVal"=w231:bool)  [unwired: 1 in]
            n109 = case shown="True" w231 {
              tunnel: [T10."Enabled" ("Disabled") T10."Disabled and Grayed Out" ("Disabled")] -> w230
              frame False {
              }
              frame True {
                n110 = property on="SingleMeas" class="Bool (strict)"("Val(Sgnl)"=FALSE ("Value (Signaling)")) -> ()  [unwired: 2 in, 2 out]
              }
            }
            n111 = property on="SingleMeas" class="Bool (strict)"("DisabledEnum"=w230) -> ()  [unwired: 2 in, 2 out]
          }
          event Value Change {
            n112 = event-data() -> ("NewVal"=w243:T6)  [unwired: 1 in]
            n113 = call "UserInput2SPCDataCluster.vi"("UserInput_In"=w243, "SPCData_In"=w244) -> ("SPCData_Out"=w242:T2)  [unwired: 9 in]
            n114 = call "SPC_set_parameters.vi"("SPCdata In"=w242, "Error In"=w247, "Module No."=w246, "DLL Path"=w245) -> ("Error Out"=w250:errorcluster, "Module No"=w249:i16, "DLL Path"=w251:path, "SPCdata Out"=w235:T2)  [unwired: 4 in]
            n115 = call "SPCDataCluster2UserInput.vi"("SPCdata In"=w235) -> ("UserInput Out"=w248:T6)  [unwired: 10 in]
            n116 = local write "User Input"(w248) -> ()
            n117 = Unbundle By Name(w235) -> ("tac_range"=w240:sgl, "tac_gain"=w239:i16, "adc_resolution"=w238:i16)
            n118 = Power Of 2(x=w238) -> (2^x=w237:dbl)
            n119 = Divide(x=w240, y=w239) -> (x/y=w241:sgl)
            n120 = Divide(x=w241, y=w237) -> (x/y=w236:dbl)
            n121 = property on="Data" class="WFGraph (strict)"("XScale.Multiplier"=w236) -> ()  [unwired: 2 in, 2 out]
          }
          event Value Change {
            n122 = event-data() -> ("NewVal"=w253:T4)  [unwired: 1 in]
            n123 = Bundle By Name(cluster=w263, "adc_resolution"=w253) -> (w264:T2)
            n124 = call "SPC_set_parameters.vi"("SPCdata In"=w264, "Error In"=w267, "Module No."=w266, "DLL Path"=w265) -> ("Error Out"=w262:errorcluster, "Module No"=w259:i16, "DLL Path"=w257:path, "SPCdata Out"=w254:T2)  [unwired: 4 in]
            n125 = call "SPCDataCluster2UserInput.vi"("SPCdata In"=w254) -> ("UserInput Out"=w268:T6)  [unwired: 10 in]
            n126 = Unbundle By Name(w254) -> ("adc_resolution"=w252:i16)
            n127 = local write "User Input"(w268) -> ()
            n128 = local read "No of Routing Channels"() -> (w256:i16)
            n129 = local write "ADC Resolution"(w252) -> ()
            n130 = call "SPC_configure_memory.vi"("No of Routing\nChannels"=w256, "Error In"=w262, "ADC Resolution [exponent]"=w252, "Module No"=w259, "DLL Path"=w257) -> ("Error Out"=w261:errorcluster, "Module No"=w260:i16, "DLL Path"=w258:path, "SPCMemConfig"=w255:T7)  [unwired: 2 in, 1 out]
            n131 = local write "SPC memory config"(w255) -> ()
          }
          event "No of Routing Channels": Value Change {
            n132 = event-data() -> ("NewVal"=w289:i16)  [unwired: 1 in]
            n133 = local read "ADC Resolution"() -> (w290:T4)
            n134 = call "SPC_configure_memory.vi"("No of Routing\nChannels"=w289, "Error In"=w286, "ADC Resolution [exponent]"=w290, "Module No"=w287, "DLL Path"=w288) -> ("Error Out"=w275:errorcluster, "Module No"=w274:i16, "DLL Path"=w273:path, "SPCMemConfig"=w291:T7)  [unwired: 2 in, 1 out]
            n135 = local write "SPC memory config"(w291) -> ()
            n136 = local read "Page"() -> (w269:i16)
            n137 = call "SPC_set_page.vi"("Error In"=w275, "Page"=w269, "Module No"=w274, "DLL Path"=w273) -> ("Error Out"=w282:errorcluster, "Page"=w276:i32, "Module No"=w281:i16, "DLL Path"=w280:path)  [unwired: 4 in]
            n138 = call "SPC_fill_memory.vi"("Fill Value"=u16 0 ("Fill value"), "Block to be Filled"=-1 ("Block to be filled"), "Error In"=w282, "Page"=w276, "Module No"=w281, "DLL Path"=w280) -> ("Error Out"=w279:errorcluster, "Module No"=w278:i16, "DLL Path"=w277:path)  [unwired: 2 in, 1 out]
            n139 = call "TestFillState.vi"("Error In"=w279, "Module No"=w278, "DLL Path"=w277) -> ("Error Out"=w270:errorcluster, "Module No"=w271:i16, "DLL Path"=w272:path)  [unwired: 6 in]
          }
          event "Page": Value Change {
            n140 = event-data() -> ("NewVal"=w298:i16)  [unwired: 1 in]
            n141 = local read "SPC memory config"() -> (w295:T7)
            n142 = Unbundle By Name(w295) -> ("Block Length"=w292:i32)
            n143 = call "SPC_set_page.vi"("Error In"=w301, "Page"=w298, "Module No"=w305, "DLL Path"=w303) -> ("Error Out"=w308:errorcluster, "Page"=w314:i32, "Module No"=w309:i16, "DLL Path"=w310:path)  [unwired: 4 in]
            n144 = call "SPC_fill_memory.vi"("Fill Value"=u16 0 ("Fill value"), "Block to be Filled"=-1 ("Block to be filled"), "Error In"=w308, "Page"=w314, "Module No"=w309, "DLL Path"=w310) -> ("Error Out"=w311:errorcluster, "Module No"=w312:i16, "DLL Path"=w313:path)  [unwired: 2 in, 1 out]
            n145 = call "TestFillState.vi"("Error In"=w311, "Module No"=w312, "DLL Path"=w313) -> ("Error Out"=w300:errorcluster, "Module No"=w304:i16, "DLL Path"=w302:path)  [unwired: 6 in]
            n146 = local read "Data"() -> (w299:u16[][])
            n147 = Initialize Array(u16 0 ("element"), w292) -> (w294:u16[])
            n148 = while {
              shift-right: [w316] -> w293
              shift-left: w299 -> [w319]
              tunnel: w298 -> [w321]
              tunnel: w294 -> [w317]
              stop <- w318 continue-if-true
              n149 = Array Size(array=w319) -> (size(s)=w322:i32[])
              n150 = Index Array(array=w322) -> (element=w320:i32)  [unwired: 1 in]
              n151 = Decrement(x=w320) -> (x-1=w315:i32)
              n152 = Greater?(x=w321, y=w315) -> (0:w318:bool)
              n153 = case shown="False" w318 {
                tunnel: w319 -> [w323 w326]
                tunnel: w317 -> [_ w325]
                tunnel: [w323 w324] -> w316
                frame False {
                }
                frame True {
                  n154 = Build Array (concatenate)(w326, w325) -> (w324:u16[][])
                }
              }
            }
            n155 = local write "Data"(w293) -> ()
          }
          event "SaveData": Value Change {
            n156 = event-data() -> ()  [unwired: 1 in, 1 out]
            n157 = local read "Data"() -> (w330:u16[][])
            n158 = case shown="\"SDT\", Default" "Save Data As" {
              tunnel: [w346 w376] -> w335
              tunnel: [w345 w375] -> w333
              tunnel: w332 -> [w344 w375]
              tunnel: w336 -> [w339 w377]
              tunnel: w331 -> [w343 w374]
              tunnel: w330 -> [w342 w368]
              tunnel: [w341 w374] -> w334
              tunnel: "SavingFolder" -> [w340 w365]
              tunnel: "Name Of File" -> [w338 w364]
              frame "SDT", Default {
                n159 = for {
                  N -> [w347]
                  tunnel: w344 -> [w356]
                  tunnel: w343 -> [w355]
                  tunnel: w342 -> [w354] mode=indexing
                  tunnel: [w353] -> w341
                  tunnel: [w357] -> w345
                  tunnel: w340 -> [w352]
                  shift-right: [w358] -> w346
                  shift-left: w339 -> [w351]
                  tunnel: w338 -> [w350]
                  i -> [w349]
                  n160 = case shown="Default" w347 {
                    tunnel: w350 -> [w359 w363]
                    tunnel: w349 -> [_ w361]
                    tunnel: [w359 w360] -> w348
                    frame 1 {
                    }
                    frame Default {
                      n161 = Format Into String(format string="_page%d" ("format string (\" (%d)\")"), initial string=w363, w361) -> (resulting string=w360:string)  [unwired: 1 in, 1 out]
                    }
                  }
                  n162 = call "SPC_save_data_to_sdtfile.vi"("Data"=w354, "Storing Path"=w352, "SDT File Name"=w348, "Error In"=w351, "Module No"=w355, "DLL Path"=w356) -> ("Error Out"=w358:errorcluster, "Module No"=w353:i16, "DLL Path"=w357:path)  [unwired: 2 in, 1 out]
                }
              }
              frame "CSV" {
                n163 = Array Size(array=w368) -> (size(s)=w369:i32[])
                n164 = Build Path(base path=w365, name or relative path=w364) -> (appended path=w366:path)
                n165 = Multiply Array Elements(1:w369) -> (0:w370:i32)
                n166 = Reshape Array(w368, w370) -> (w367:u16[])
                n167 = Decimate 1D Array(w367) -> (w373:u16[], w372:u16[])
                n168 = Join Numbers(hi=w372, lo=w373) -> ((hi.lo)=w371:u32[])
                n169 = call-poly <vilib>:"Write Delimited Spreadsheet.vi"("file path (dialog if empty)"=w366, "1D data"=w371, "error in (no error)"=w377) -> ("error out"=w376:errorcluster)  [unwired: 11 in, 1 out]
              }
            }
            n170 = flat-sequence {
              tunnel: w335 -> [_]
              frame #0 {
                n171 = local write "SaveData"(TRUE ("SaveData")) -> ()
              }
            }
          }
          event "StopVi": Value Change {
            n172 = event-data() -> ()  [unwired: 1 in, 6 out]
            n173 = local read "SaveData"() -> (w385:bool)
            n174 = case shown="False" w385 {
              tunnel: [w409 TRUE] -> w380
              frame False {
                n175 = Two Button Dialog(message="There is unsafed acquired data", 1:"Exit", 2:"Save") -> (T button?=w410:bool)
                n176 = Not(x=w410) -> (.not. x?=w409:bool)
              }
              frame True {
              }
            }
            n177 = case shown="True" w380 {
              tunnel: w382 -> [w388 w398]
              tunnel: w384 -> [w387 w397]
              tunnel: [w388 w396] -> w383
              tunnel: [w387 w394] -> w381
              frame False {
              }
              frame True {
                n178 = call "SPC_close.vi"("Error In"=w397, "DLL Path"=w398) -> ("Error Out"=w395:errorcluster, "DLL Path"=w396:path)  [unwired: 8 in]
                n179 = property class="App"() -> ("App.Name"=w393:string)  [unwired: 2 in, 2 out]
                n180 = Not Equal?(x=w393, y="LabVIEW.exe") -> (x != y?=w391:bool)
                n181 = local write "RepeatMeas"(FALSE ("SingleMeas")) -> ()
                n182 = case shown="False" w391 {
                  selector: w391 -> [_ w403]
                  tunnel: w395 -> [w400 w405]
                  tunnel: [w400 w404] -> w394
                  frame False {
                    n183 = Stop(stop? (T)=TRUE) -> ()
                  }
                  frame True {
                    n184 = Call Chain() -> (call chain=w402:string[])
                    n185 = Index Array(array=w402) -> (element=w401:string)  [unwired: 1 in]
                    n186 = Open VI Reference(vi path=w401, error in (no error)=w405) -> (vi reference=w407:refnum<vi>, error out=w406:errorcluster)  [unwired: 4 in]
                    n187 = invoke class="VI" method="FP.Close"(reference=w407, error in=w406) -> (error out=w404:errorcluster)  [unwired: 1 in, 2 out]
                    n188 = flat-sequence {
                      tunnel: w404 -> [_]
                      tunnel: w403 -> [w408]
                      frame #0 {
                        n189 = Quit LabVIEW(quit? (T)=w408) -> ()
                      }
                    }
                  }
                }
                n190 = property on="SingleMeas" class="Bool (strict)"("DisabledEnum"=T10."Enabled" ("Disabled")) -> ()  [unwired: 2 in, 2 out]
              }
            }
          }
        }
      }
      frame Error {
        w415 = T10."Enabled" ("Disabled")
        w416 = FALSE ("StartMeas")
        n191 = call <vilib>:"Simple Error Handler.vi"("error in (no error)"=w420) -> ()  [unwired: 4 in, 5 out]
        n192 = local write "SingleMeas"(w416) -> ()
        n193 = local write "RepeatMeas"(w416) -> ()
        n194 = property on="RepeatMeas" class="Bool (strict)"("DisabledEnum"=w415) -> ()  [unwired: 2 in, 2 out]
        n195 = property on="SingleMeas" class="Bool (strict)"("DisabledEnum"=w415) -> ()  [unwired: 2 in, 2 out]
      }
    }
  }
